vi "e.gate Example - HighSpeedPort Online Communication.vi"(8 "Fehler (Eingang, kein Fehler)":errorcluster, 11 "IP Address":string) -> (0 "error out":errorcluster)   [LabVIEW 2016]
uses:
  e.gate Configuration.ctl
  e.gate Channel Data.ctl
  e.gate Data Type.ctl
  e.gate Protocol Type.ctl
  e.gate Module  Data.ctl
  e.gateHSP_DLLhandle.ctl
panel:
  out "e.gate Configuration Out":T1
  in  "delay":u32
  out "IP Address":string
  out "Value 2":dbl[](graph)
  in  "ValueArray":dbl[](array[numeric])
  in  "WriteCount":i32
  in  "Write Index":i32
  in  "ReadCount":i32
  in  "ReadIndex":i32
  in  "Stop":bool
  # "EXAMPLE - HighSpeedPort online communication"
  # "Write Channel"
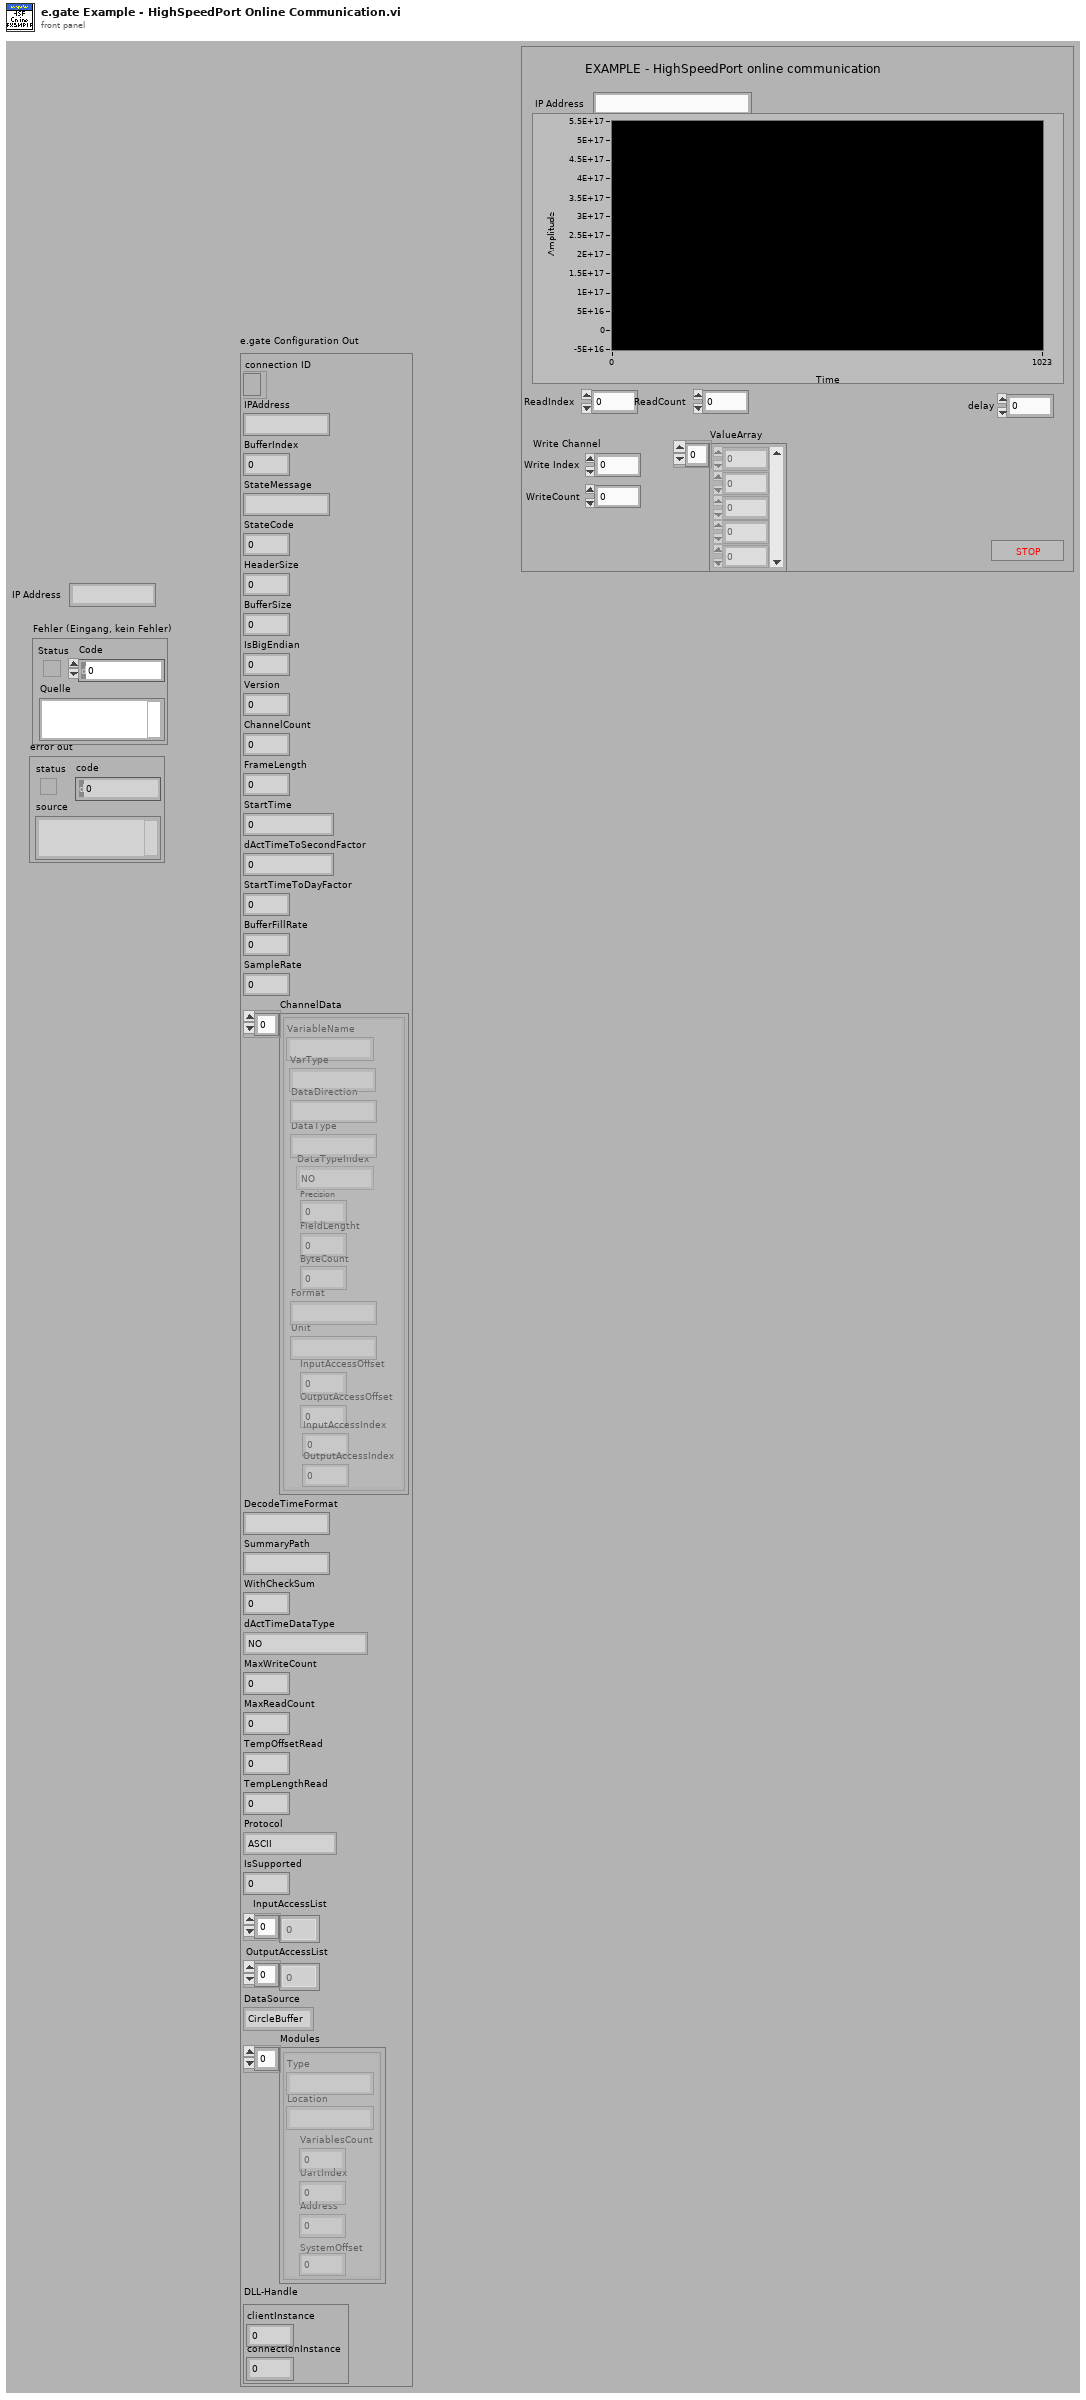
[diagram p1: front panel]
types:
  T1 = typedef "e.gate Configuration.ctl" = cluster{"connection ID":refnum<k5>, "IPAddress":string, "BufferIndex":i32, "StateMessage":string, "StateCode":i8, "HeaderSize":i32, "BufferSize":i32, "IsBigEndian":i32, "Version":i32, "ChannelCount":i32, "FrameLength":i32, "StartTime":dbl, "dActTimeToSecondFactor":dbl, "StartTimeToDayFactor":dbl, "BufferFillRate":dbl, "SampleRate":dbl, "ChannelData":T2[], "DecodeTimeFormat":string, "SummaryPath":string, "WithCheckSum":i32, "dActTimeDataType":T3, "MaxWriteCount":i32, "MaxReadCount":i32, "TempOffsetRead":i32, "TempLengthRead":i32, "Protocol":T4, "IsSupported":i32, "InputAccessList":i32[], "OutputAccessList":i32[], "DataSource":enum16{"CircleBuffer", "test.con Logger", "test.con Archive"}, "Modules":T5[], "DLL-Handle":T6}
  T2 = typedef "e.gate Channel Data.ctl" = cluster{"VariableName":string, "DataDirection":string, "DataType":string, "DataTypeIndex":T3, "Precision":i16, "FieldLengtht":i16, "ByteCount":i32, "Format":string, "Unit":string, "InputAccessOffset":i32, "OutputAccessOffset":i16, "InputAccessIndex":i16, "OutputAccessIndex":i16, "VarType":string}
  T3 = typedef "e.gate Data Type.ctl" = enum16{"NO", "BOOL", "SINT8", "USINT8", "SINT16", "USINT16", "SINT32", "USINT32", "FLOAT", "SET8", "SET16", "SET32", "DOUBLE", "SINT64", "USINT64", "SET64"}
  T4 = typedef "e.gate Protocol Type.ctl" = enum16{"ASCII", "HighspeedPort Online", "HighspeedPort Buffer", "eGateHighspeedPortDLL "}
  T5 = typedef "e.gate Module  Data.ctl" = cluster{"Type":string, "Location":string, "VariablesCount":i16, "UartIndex":i16, "Address":i16, "SystemOffset":i16}
  T6 = typedef "e.gateHSP_DLLhandle.ctl" = cluster{"clientInstance":i32, "connectionInstance":i32}
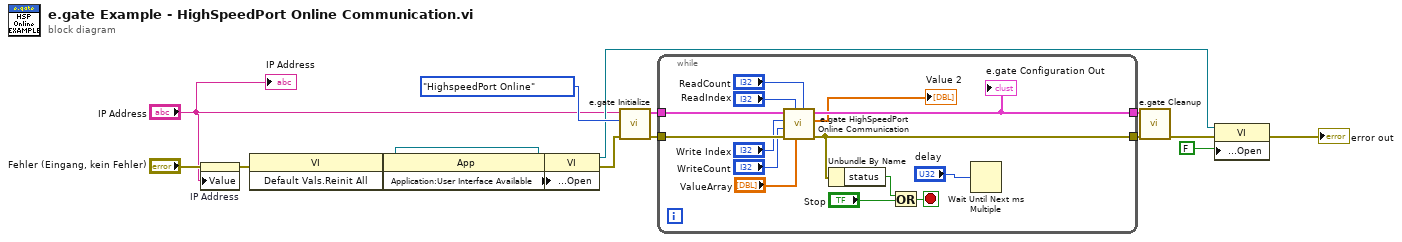
[diagram p0: block diagram]
diagram:
  n1 = property on="IP Address" class="Str"(error in="Fehler (Eingang, kein Fehler)", "Value"="IP Address") -> (error out=w2:errorcluster)  [unwired: 1 in, 1 out]
  n2 = invoke class="VI" method="Default Vals.Reinit All"(error in=w2) -> (reference out=w12:refnum<vi>, error out=w10:errorcluster)  [unwired: 2 in, 1 out]
  n3 = property class="App"(error in=w10) -> (error out=w9:errorcluster, "Application:User Interface Available"=w11:bool)  [unwired: 1 in, 1 out]
  n4 = property class="VI"(reference=w12, error in=w9, "Front Panel.Open"=w11) -> (reference out=w4:refnum<vi>, error out=w8:errorcluster)
  n5 = call "e.gate Initialize.vi"("error in (no error)"=w8, "Protocol"=e.gate_Protocol_Type."HighspeedPort Online", "IP Address"="IP Address") -> ("error out"=w15:errorcluster, "e.gate Configuration"=w17:T1)  [unwired: 1 in, 6 out]
  n6 = while {
    tunnel: w17 -> [w31]
    tunnel: [w30] -> w16
    tunnel: w15 -> [w29]
    tunnel: [w28] -> w14
    stop <- w27 stop-if-true
    n7 = call "e.gate HighSpeedPort Online Communication.vi"("ReadCount"="ReadCount", "ValueArray"="ValueArray", "ReadIndex"="ReadIndex", "error in (no error)"=w29, "WriteCount"="WriteCount", "WriteIndex"="Write Index", "e.gate Configuration In"=w31) -> ("error out"=w28:errorcluster, "Value"=→"Value 2":dbl[], "e.gate Configuration Out"=w30:T1)  [unwired: 2 out]
    "e.gate Configuration Out" <- w30
    n8 = Unbundle By Name(w28) -> ("status"=w26:bool)
    n9 = Or(x=w26, y="Stop") -> (x .or. y?=w27:bool)
    n10 = Wait Until Next ms Multiple(millisecond multiple="delay") -> ()  [unwired: 1 out]
  }
  n11 = call "e.gate Cleanup.vi"("error in (no error)"=w14, "e.gate Configuration"=w16) -> ("error out"=w7:errorcluster)  [unwired: 9 out]
  n12 = property class="VI"(reference=w4, error in=w7, "Front Panel.Open"=FALSE ("Frontpanel-Fenster:Öffnen")) -> (error out=→"error out":errorcluster)  [unwired: 1 out]
  "IP Address" <- "IP Address"
